vi "NormaliseHeight.vi"(5 "NormaliseHeight?":bool, 7 "Zref":dbl, 11 "Value-Z Cluster In":cluster{"Array":dbl[], "Array":dbl[]}) -> (3 "Value-Z Cluster Out":cluster{"Array":dbl[], "Array":dbl[]})   [LabVIEW 2021]
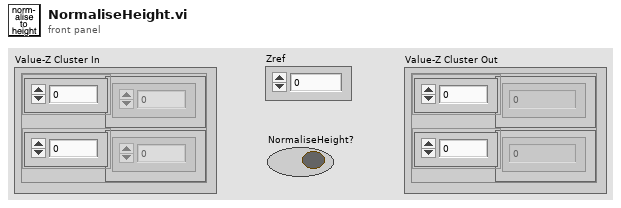
[diagram p1: front panel]
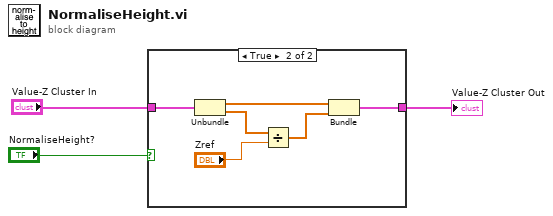
[diagram p0: block diagram]
diagram:
  n1 = case shown="True" "NormaliseHeight?" {
    tunnel: "Value-Z Cluster In" -> [w4 w10]
    tunnel: [w4 w5] -> w2
    frame False {
    }
    frame True {
      n2 = Unbundle(w10) -> ("Array"=w9:dbl[], "Array"=w8:dbl[])
      n3 = Divide(x=w8, y="Zref") -> (x/y=w7:dbl[])
      n4 = Bundle("Array"=w9, w7) -> (w5:cluster{"Array":dbl[], dbl[]})  [unwired: 1 in]
    }
  }
  "Value-Z Cluster Out" <- w2
